vi "prepare tiff right.vi"(2 "z":i32, 3 "y":i32, 4 "x":i32, 5 "file path":path) -> (0 "error out":errorcluster, 1 "refnum tif":refnum<file>)   [LabVIEW 2012]
panel:
  out "x*y":i32
  out "IFDend":u32
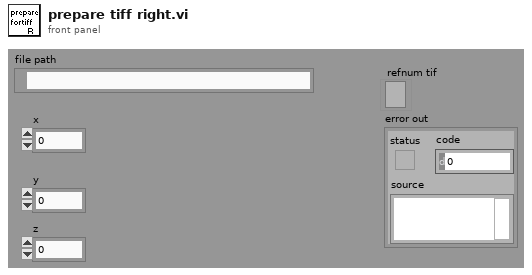
[diagram p1: front panel]
types:
  T1 = enum16{"open", "replace", "create", "open or create", "replace or create", "replace or create with confirmation"}
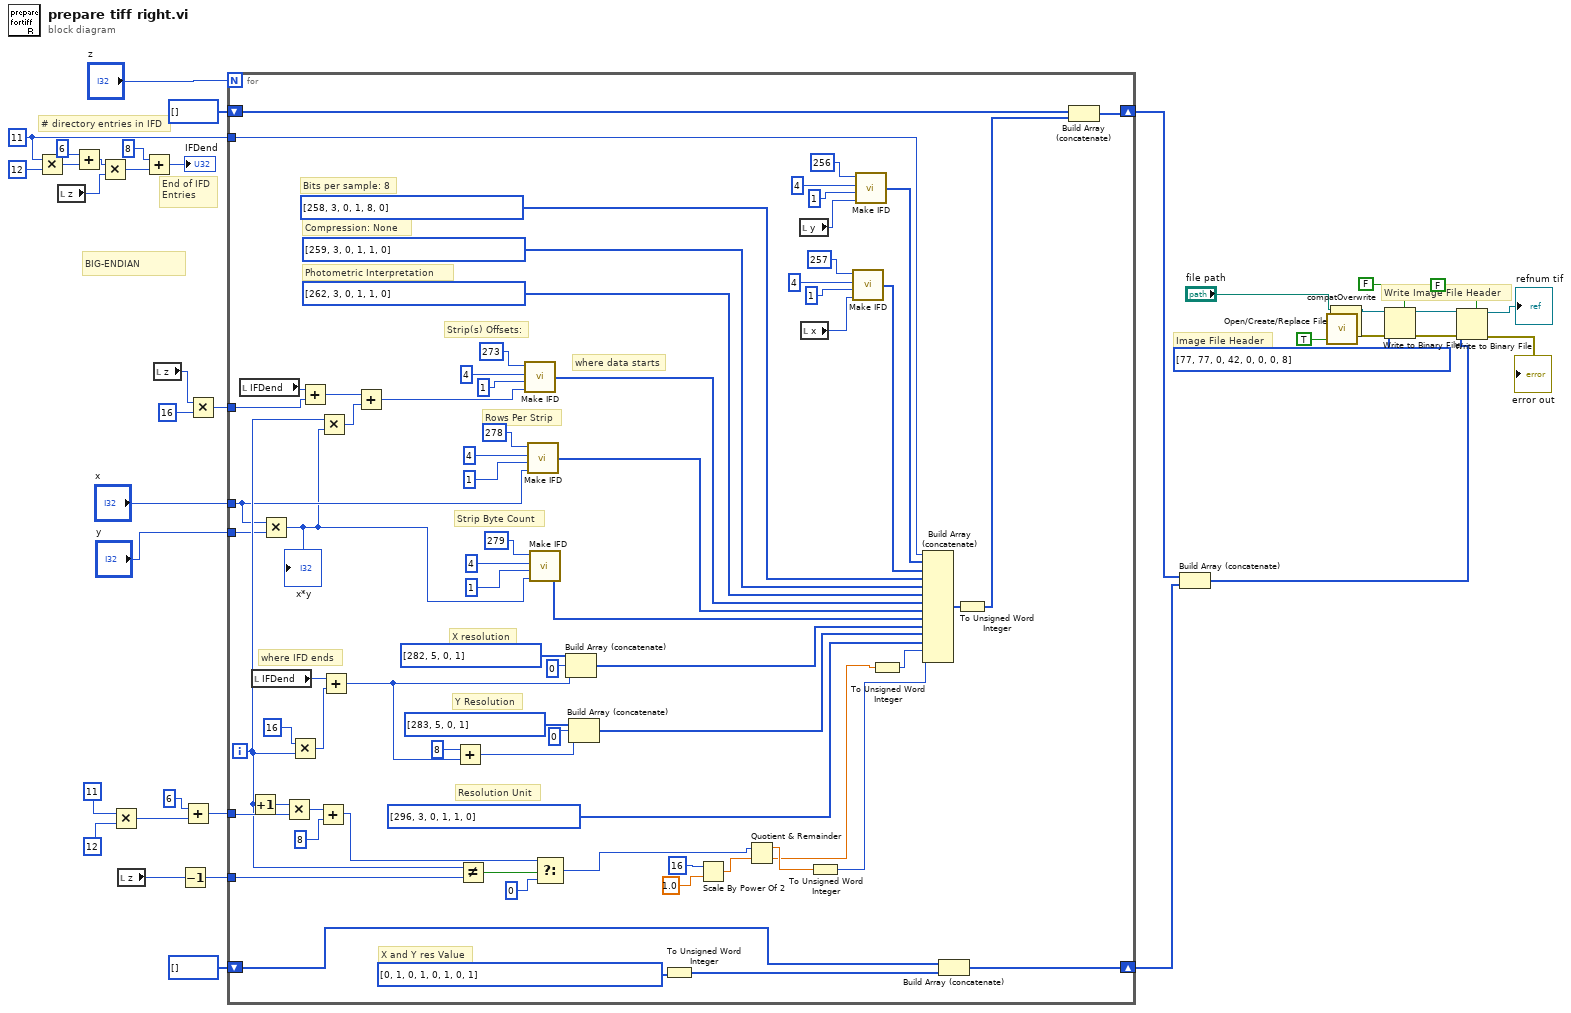
[diagram p0: block diagram]
diagram:
  w31 = u16 11
  # "Image File Header"
  # "Write Image File Header"
  # "End of IFD\nEntries"
  # "# directory entries in IFD"
  # "BIG-ENDIAN"
  n1 = Multiply(x=w31, y=u16 12) -> (x*y=w30:u16)
  n2 = local read "z"() -> (w21:i32)
  n3 = Add(x=u16 6, y=w30) -> (x+y=w24:u16)
  n4 = Multiply(x=w24, y=w21) -> (x*y=w36:i32)
  n5 = Multiply(x=11, y=12) -> (x*y=w26:i32)
  n6 = local read "z"() -> (w19:i32)
  n7 = Add(x=8, y=w36) -> (x+y=→"IFDend":i32)
  n8 = local read "z"() -> (w20:i32)
  n9 = Decrement(x=w19) -> (x-1=w22:i32)
  n10 = Add(x=u16 6, y=w26) -> (x+y=w25:i32)
  n11 = Multiply(x=w20, y=16) -> (x*y=w32:i32)
  n12 = for {
    N: "z" -> [_]
    shift-right: [w65] -> w17
    shift-left: u16[] [] -> [w78]
    shift-right: [w75] -> w16
    shift-left: u16[] [] -> [w74]
    tunnel: w31 -> [w73]
    tunnel: w32 -> [w68]
    tunnel: w25 -> [w61]
    tunnel: w22 -> [w57]
    tunnel: "x" -> [w48]
    tunnel: "y" -> [w47]
    i -> [w56]
    # "where IFD ends"
    # "where data starts"
    # "X and Y res Value"
    # "Resolution Unit"
    # "Y Resolution"
    # "X resolution"
    # "Bits per sample: 8"
    # "Strip Byte Count"
    # "Rows Per Strip"
    # "Strip(s) Offsets:"
    # "Photometric Interpretation"
    # "Compression: None"
    n13 = local read "IFDend"() -> (w93:u32)
    n14 = Increment(x=w56) -> (x+1=w51:i32)
    n15 = local read "IFDend"() -> (w72:u32)
    n16 = Multiply(x=w48, y=w47) -> (x*y=w46:i32)
    "x*y" <- w46
    n17 = Multiply(x=w51, y=w61) -> (x*y=w60:i32)
    n18 = Multiply(x=16, y=w56) -> (x*y=w70:i32)
    n19 = Add(x=w93, y=w68) -> (x+y=w67:u32)
    n20 = Add(x=w60, y=8) -> (x+y=w58:i32)
    n21 = Multiply(x=w56, y=w46) -> (x*y=w66:i32)
    n22 = Add(x=w72, y=w70) -> (x+y=w71:u32)
    n23 = Add(x=w67, y=w66) -> (x+y=w64:u32)
    n24 = Add(x=u32 8, y=w71) -> (x+y=w63:u32)
    n25 = Not Equal?(x=w56, y=w57) -> (x != y?=w55:bool)
    n26 = call "Make IFD.vi"("Value/Offset"=w64, "Count"=u32 1, "TYPE"=u16 4, "TAG"=u16 273) -> ("IFD entry"=w87:u16[])
    n27 = call "Make IFD.vi"("Value/Offset"=w48, "Count"=u32 1, "TYPE"=u16 4, "TAG"=u16 278) -> ("IFD entry"=w86:u16[])
    n28 = call "Make IFD.vi"("Value/Offset"=w46, "Count"=u32 1, "TYPE"=u16 4, "TAG"=u16 279) -> ("IFD entry"=w85:u16[])
    n29 = Select(t=w58, s=w55, f=u16 0) -> (s? t:f=w42:i32)
    n30 = Build Array (concatenate)(u16[] [282, 5, 0, 1], 0, w71) -> (w84:u32[])
    n31 = Build Array (concatenate)(u16[] [283, 5, 0, 1], 0, w63) -> (w83:u32[])
    n32 = To Unsigned Word Integer(number=u16[] [0, 1, 0, 1, 0, 1, 0, 1]) -> (unsigned 16bit integer=w76:u16[])
    n33 = Scale By Power Of 2(n=16, x=1.0) -> (x*2^n=w43:dbl)
    n34 = Quotient & Remainder(x=w42, y=w43) -> (x-y*floor(x/y)=w41:dbl, floor(x/y)=w40:dbl)
    n35 = local read "y"() -> (w49:i32)
    n36 = local read "x"() -> (w50:i32)
    n37 = To Unsigned Word Integer(number=w41) -> (unsigned 16bit integer=w53:u16)
    n38 = call "Make IFD.vi"("Value/Offset"=w50, "Count"=u32 1, "TYPE"=u16 4, "TAG"=u16 257) -> ("IFD entry"=w91:u16[])
    n39 = call "Make IFD.vi"("Value/Offset"=w49, "Count"=u32 1, "TYPE"=u16 4, "TAG"=u16 256) -> ("IFD entry"=w92:u16[])
    n40 = To Unsigned Word Integer(number=w40) -> (unsigned 16bit integer=w52:u16)
    n41 = Build Array (concatenate)(w73, w92, w91, u16[] [258, 3, 0, 1, 8, 0], u16[] [259, 3, 0, 1, 1, 0], u16[] [262, 3, 0, 1, 1, 0], w87, w86, w85, w84, w83, u16[] [296, 3, 0, 1, 1, 0], w52, w53) -> (w81:u32[])
    n42 = Build Array (concatenate)(w74, w76) -> (w75:u16[])
    n43 = To Unsigned Word Integer(number=w81) -> (unsigned 16bit integer=w62:u16[])
    n44 = Build Array (concatenate)(w78, w62) -> (w65:u16[])
  }
  n45 = Build Array (concatenate)(w17, w16) -> (w8:u16[])
  n46 = call <vilib>:"compatOverwrite.vi"("overwrite (F)"=TRUE) -> ("overwrite?"=w1:T1)
  n47 = Open/Create/Replace File(file path (use dialog)="file path", operation (0:open)=w1) -> (refnum out=w9:refnum<file>, error out=w12:errorcluster)  [unwired: 4 in, 1 out]
  n48 = Write to Binary File(file (use dialog)=w9, data=u8[] [77, 77, 0, 42, 0, 0, 0, 8], error in=w12, 5:FALSE ("prepend array or string size? (T)")) -> (refnum out=w10:refnum<file>, error out=w11:errorcluster)  [unwired: 2 in, 1 out]
  n49 = Write to Binary File(file (use dialog)=w10, data=w8, error in=w11, 5:FALSE ("prepend array or string size? (T)")) -> (refnum out=→"refnum tif":refnum<file>, error out=→"error out":errorcluster)  [unwired: 2 in, 1 out]
